vi "Stop all tasks.vi"(8 "error in":errorcluster, 11 "Task list":T1) -> (0 "error out":errorcluster)   [LabVIEW 2018]
uses:
  <vilib>/vision/driver/NI_Vision_Acquisition_Software.lvlib
  typedef/Task list.ctl
  <vilib>/userDefined/High Color/IMAQdx.ctl
  <vilib>/vision/Image Controls.llb/IMAQ Image.ctl
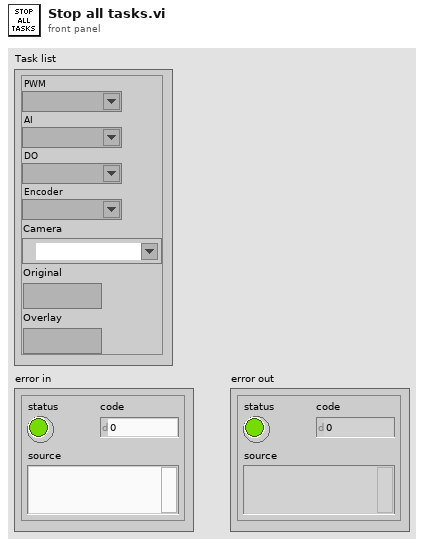
[diagram p1: front panel]
types:
  T1 = typedef "Task list.ctl" = cluster{"PWM":refnum<k21>, "AI":refnum<k21>, "DO":refnum<k21>, "Encoder":refnum<k21>, "Camera":T2, "Original":T3, "Overlay":T3}
  T2 = typedef "IMAQdx.ctl" = refnum<k21>
  T3 = typedef "IMAQ Image.ctl" = refnum<image>
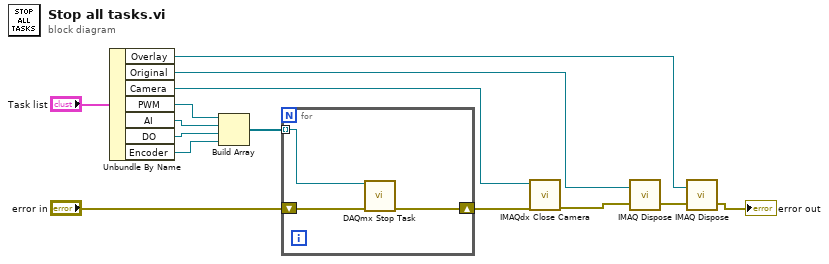
[diagram p0: block diagram]
diagram:
  n1 = Unbundle By Name("Task list") -> ("Overlay"=w1:T3, "Original"=w4:T3, "Camera"=w5:T2, "PWM"=w12:refnum<k21>, "AI"=w11:refnum<k21>, "DO"=w10:refnum<k21>, "Encoder"=w9:refnum<k21>)
  n2 = Build Array(w12, w11, w10, w9) -> (w8:refnum<k21>[])
  n3 = for {
    shift-right: [w16] -> w7
    shift-left: "error in" -> [w17]
    tunnel: w8 -> [w15] mode=indexing
    n4 = call <vilib>:"DAQmx Stop Task.vi"("task/channels in"=w15, "error in"=w17) -> ("error out"=w16:errorcluster)  [unwired: 12 in, 1 out]
  }
  n5 = call <vilib>:"IMAQdx Close Camera.vi"("error in"=w7, "Session In"=w5) -> ("error out"=w6:errorcluster)  [unwired: 9 in]
  n6 = call "IMAQ Dispose"("Image"=w4, "error in (no error)"=w6) -> ("error out"=w3:errorcluster)  [unwired: 4 in]
  n7 = call "IMAQ Dispose"("Image"=w1, "error in (no error)"=w3) -> ("error out"=→"error out":errorcluster)  [unwired: 4 in]
